vi "Read_Write Temp_Humi TCP Example.vi"() -> ()   [LabVIEW 2021, in "Environment Chamber.lvlib" / "Climatic Chamber.lvlib"]
doc: "Example to <b>monitor</b> the actual <b>temperature and humidity</b>.\nAnd to <b>conifgure</B> the <b>temperature and humidity settings</b>.\nAfter the configuration is sent to the chamber, the chamber is then turned on."
uses:
  Climatic Chamber.lvlib
  Private/Type Defs/Operation_Stop Mode Enum.ctl
panel:
  in  "lower limit":dbl
  in  "upper limit":dbl=80.0
  in  "lower limit":dbl
  in  "upper limit":dbl=80.0
  in  "Humidity setpoint":dbl=50.0
  in  "Temperature setpoint":dbl=40.0
  in  "Update Chamber (4)":bool
  in  "IP Address":string="0.0.0.0"
  out "New Data":bool
  in  "stop":bool
  out "Humidity":dbl(slide) scale=0.0..100.0
  out "Temperature":dbl(slide) scale=0.0..100.0
  out "Instrument Firmware Revision":string
  # "1. Enter IP Address (dot\nnotation) that matches the\nsettings in your chamber\n\n2. Run the VI\n\n3. Configure the Temperature\nand Humidity settings\n\n4. Update the Chamber"
  # "IP Address (1)"
  # "Configuration (3)"
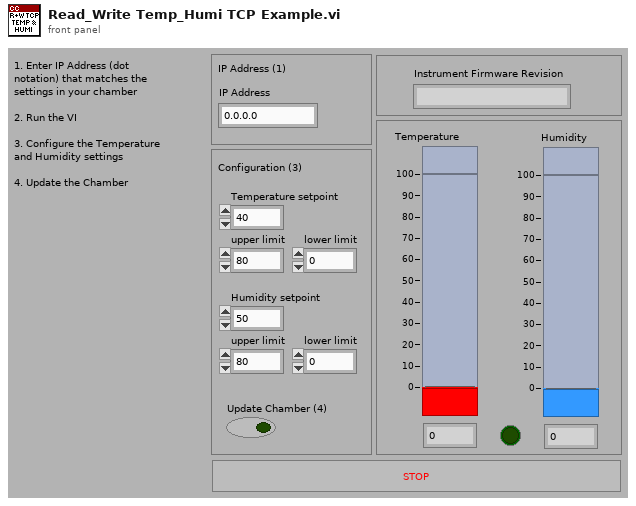
[diagram p1: front panel]
types:
  T1 = typedef "Environment Chamber.lvlib/Climatic Chamber.lvlib/Operation_Stop Mode Enum.ctl" = enum16{"RUN", "CONSTANT", "STANDBY", "OFF"}
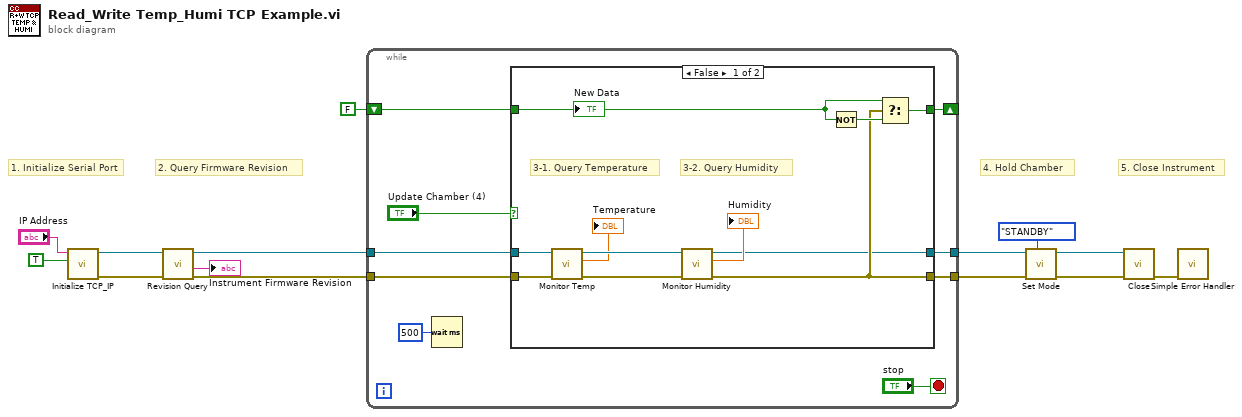
[diagram p0: block diagram]
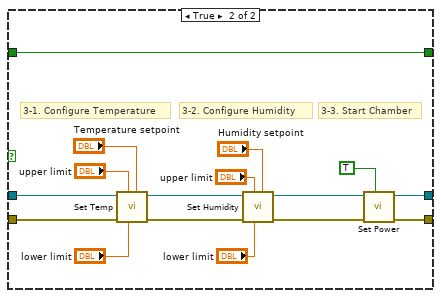
[diagram p2: hidden frame]
diagram:
  # "4. Hold Chamber"
  # "5. Close Instrument"
  # "2. Query Firmware Revision"
  # "1. Initialize Serial Port"
  n1 = call "Initialize TCP_IP.vi"("ID Query (True)"=TRUE, "TCP/IP Address"="IP Address") -> ("error out"=w12:errorcluster, "VISA resource name out"=w13:refnum<visa-resource-name>)  [unwired: 8 in]
  n2 = call "Revision Query.vi"("error in (no error)"=w12, "VISA resource name"=w13) -> ("error out"=w11:errorcluster, "Instrument Firmware Revision"=→"Instrument Firmware Revision":string, "VISA resource name out"=w10:refnum<visa-resource-name>)  [unwired: 6 in, 1 out]
  n3 = while {
    tunnel: w11 -> [w23]
    tunnel: w10 -> [w22]
    tunnel: [w21] -> w4
    tunnel: [w20] -> w5
    shift-right: [w15] -> _
    shift-left: FALSE -> [w16]
    stop <- "stop" stop-if-true
    n4 = Wait (ms)(milliseconds to wait=u32 500) -> ()  [unwired: 1 out]
    n5 = case shown="False" "Update Chamber (4)" {
      tunnel: w23 -> [w34 w49]
      tunnel: w22 -> [w33 w50]
      tunnel: [w25 w45] -> w21
      tunnel: [w24 w43] -> w20
      tunnel: w16 -> [w26 w41]
      tunnel: [w28 w41] -> w15
      frame False {
        # "3-2. Query Humidity"
        # "3-1. Query Temperature"
        n6 = call "Monitor Temp.vi"("error in (no error)"=w34, "VISA resource name"=w33) -> ("error out"=w32:errorcluster, "measured temp"=→"Temperature":dbl, "VISA resource name out"=w31:refnum<visa-resource-name>)  [unwired: 4 in, 3 out]
        n7 = call "Monitor Humidity.vi"("error in (no error)"=w32, "VISA resource name"=w31) -> ("error out"=w25:errorcluster, "measured humidity"=→"Humidity":dbl, "VISA resource name out"=w24:refnum<visa-resource-name>)  [unwired: 4 in, 3 out]
        n8 = Not(x=w26) -> (.not. x?=w27:bool)
        n9 = Select(t=w26, s=w25, f=w27) -> (s? t:f=w28:bool)
        "New Data" <- w26
      }
      frame True {
        # "3-3. Start Chamber"
        # "3-2. Configure Humidity"
        # "3-1. Configure Temperature"
        n10 = call "Set Temp.vi"("Temp"="Temperature setpoint", "Lower Limit"="lower limit", "Upper Limit"="upper limit", "error in (no error)"=w49, "VISA resource name"=w50) -> ("error out"=w47:errorcluster, "VISA resource name out"=w48:refnum<visa-resource-name>)  [unwired: 5 in]
        n11 = call "Set Humidity.vi"("Humidity"="Humidity setpoint", "Lower Limit"="lower limit", "Upper Limit"="upper limit", "error in (no error)"=w47, "VISA resource name"=w48) -> ("error out"=w46:errorcluster, "VISA resource name out"=w44:refnum<visa-resource-name>)  [unwired: 5 in]
        n12 = call "Set Power.vi"("Power (On/Off)"=TRUE, "error in (no error)"=w46, "VISA resource name"=w44) -> ("error out"=w45:errorcluster, "VISA resource name out"=w43:refnum<visa-resource-name>)  [unwired: 7 in]
      }
    }
  }
  n13 = call "Set Mode.vi"("Operation Mode"=Operation_Stop_Mode_Enum."STANDBY", "error in (no error)"=w4, "VISA resource name"=w5) -> ("error out"=w3:errorcluster, "VISA resource name out"=w2:refnum<visa-resource-name>)  [unwired: 7 in]
  n14 = call "Close.vi"("error in (no error)"=w3, "VISA resource name"=w2) -> ("error out"=w8:errorcluster)  [unwired: 9 in]
  n15 = call <vilib>:"Simple Error Handler.vi"("error in (no error)"=w8) -> ()  [unwired: 4 in, 5 out]
